vi "Configure CONT.vi"(0 "VISA resource name":refnum<visa-resource-name>, 1 "Test Time (s)":string, 2 "Min Cont Limit (ohm)":string, 3 "Max Cont Limit (ohm)":string, 4 "Command Terminator":bool=TRUE, 5 "error in (no error)":errorcluster) -> (14 "VISA resource name out":refnum<visa-resource-name>, 15 "Command Output":string, 17 "Error Message":string, 18 "Error Code":i32, 19 "error out":errorcluster)   [LabVIEW 2010, in "VITREK V7X.lvlib"]
doc: "Configures the <b>CONT</b> input.\n\n<b>Note:</b> please refer to the instrument manual for the <b>CONT</b> input specification."
uses:
  VITREK V7X.lvlib
panel:
  # "Yes\n\nNo"
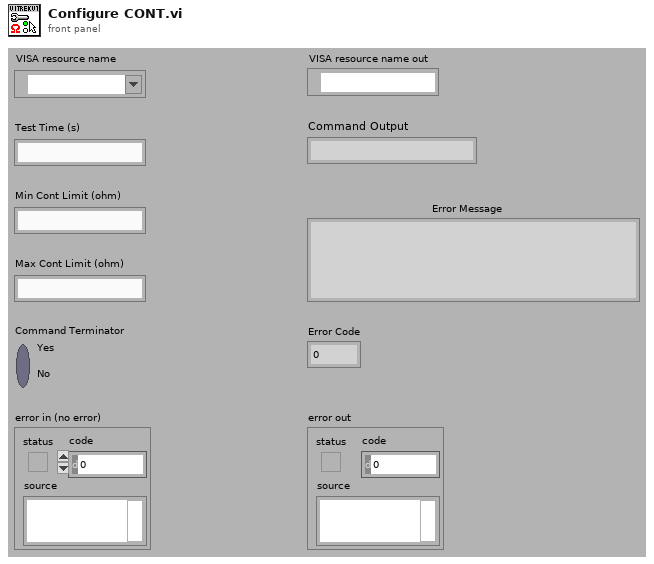
[diagram p1: front panel]
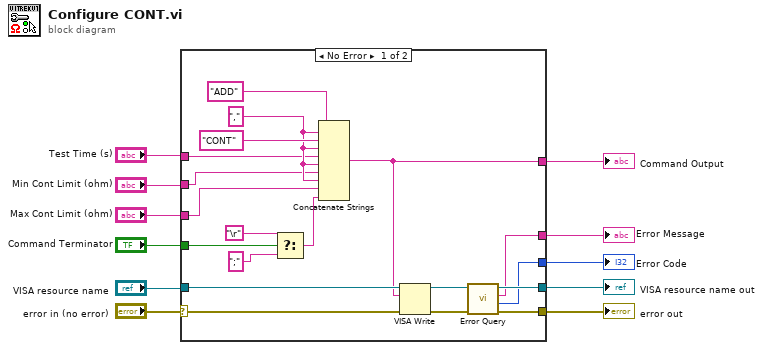
[diagram p0: block diagram]
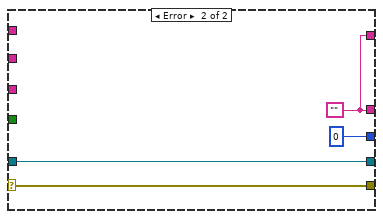
[diagram p2: hidden frame]
diagram:
  n1 = case shown="No Error" "error in (no error)" {
    selector: "error in (no error)" -> [w25 w33]
    tunnel: "VISA resource name" -> [w30 w34]
    tunnel: [w23 w31] -> w10
    tunnel: [w27 w34] -> w9
    tunnel: [w26 w33] -> w8
    tunnel: "Test Time (s)" -> [w16 _]
    tunnel: "Min Cont Limit (ohm)" -> [w15 _]
    tunnel: "Max Cont Limit (ohm)" -> [w14 _]
    tunnel: "Command Terminator" -> [w22 _]
    tunnel: [w13 0 ("Error Code")] -> w2
    tunnel: [w12 w31] -> w1
    frame No Error {
      w18 = ","
      n2 = Select(t="\r", s=w22, f=";") -> (s? t:f=w17:string)
      n3 = Concatenate Strings("ADD", w18, "CONT", w18, w16, w18, w15, w18, w14, w17) -> (w23:string)
      n4 = VISA Write(VISA resource name=w30, write buffer=w23, error in (no error)=w25) -> (VISA resource name out=w29:refnum<visa-resource-name>, error out=w28:errorcluster)  [unwired: 1 out]
      n5 = call "Error Query.vi"("error in (no error)"=w28, "VISA resource name"=w29) -> ("error out"=w26:errorcluster, "Error Code"=w13:i32, "Error Message"=w12:string, "VISA resource name out"=w27:refnum<visa-resource-name>)  [unwired: 6 in]
    }
    frame Error {
      w31 = ""
    }
  }
  "VISA resource name out" <- w9
  "error out" <- w8
  "Command Output" <- w10
  "Error Code" <- w2
  "Error Message" <- w1
